vi "getLogDir.vi"() -> (3 "dirLog":path)   [LabVIEW 2018]
doc: "Get the log directory."
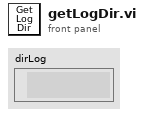
[diagram p1: front panel]
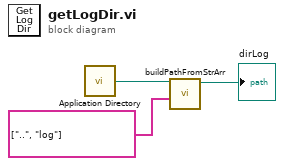
[diagram p0: block diagram]
diagram:
  n1 = call <vilib>:"Application Directory.vi"() -> ("Application Directory"=w3:path)
  n2 = call "buildPathFromStrArr.vi"("String Array"=string[] ["..", "log"], "Root Path"=w3) -> ("Absolute Path"=→"dirLog":path)  [unwired: 9 in]
